vi "Steering Motor Control Test.vi"() -> ()   [LabVIEW 2010]
uses:
  Motor Output Global.vi
  Motor Encoder Global.vi
panel:
  in  "Steering Position Target":i32
  in  "Steering Enable":bool
  out "Steering Encoder":i32
  in  "Steering Proportional Control Feedback Gain":fxp<+/-,20,5>
  in  "stop":bool
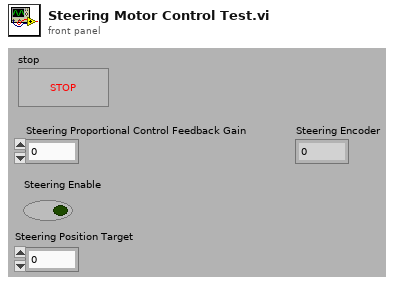
[diagram p1: front panel]
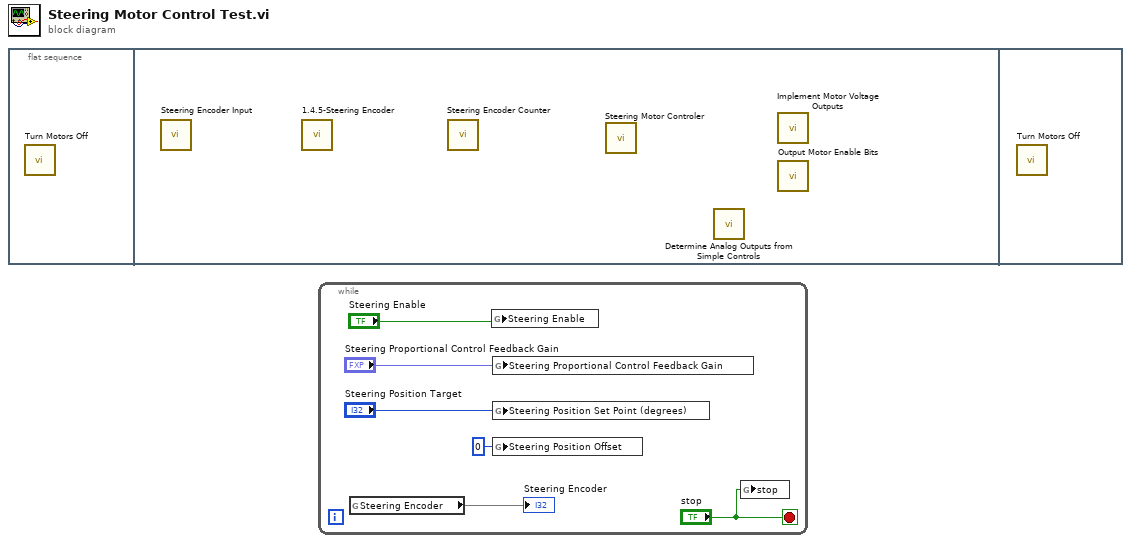
[diagram p0: block diagram]
diagram:
  n1 = flat-sequence {
    frame #0 {
      n2 = call "Turn Motors Off.vi"() -> ()  [unwired: 1 in]
    }
    frame #1 {
      n3 = call "Steering Encoder Input.vi"() -> ()  [unwired: 1 in]
      n4 = call "1.4.5-Steering Encoder.vi"() -> ()  [unwired: 1 in]
      n5 = call "Steering Encoder Counter.vi"() -> ()  [unwired: 1 in]
      n6 = call "Steering Motor Controler.vi"() -> ()  [unwired: 1 in]
      n7 = call "Determine Analog Outputs from Simple Controls.vi"() -> ()  [unwired: 1 in]
      n8 = call "Implement Motor Voltage Outputs.vi"() -> ()  [unwired: 1 in]
      n9 = call "Output Motor Enable Bits.vi"() -> ()  [unwired: 1 in]
    }
    frame #2 {
      n10 = call "Turn Motors Off.vi"() -> ()  [unwired: 1 in]
    }
  }
  n11 = while {
    stop <- "stop" stop-if-true
    n12 = global read "Motor Encoder Global.vi" "Steering Encoder"() -> (→"Steering Encoder")
    n13 = global write "Motor Output Global.vi" "Steering Enable"("Steering Enable") -> ()
    n14 = global write "Motor Encoder Global.vi" "Steering Proportional Control Feedback Gain"("Steering Proportional Control Feedback Gain") -> ()
    n15 = global write "Motor Encoder Global.vi" "Steering Position Set Point (degrees)"("Steering Position Target") -> ()
    n16 = global write "Motor Encoder Global.vi" "Steering Position Offset"(0 ("Steering Position Offset")) -> ()
    n17 = global write "Motor Encoder Global.vi" "stop"("stop") -> ()
  }
